vi "Read_SystemDevices_Values.vi"(8 "error in (no error)":errorcluster) -> (0 "error out":errorcluster)   [LabVIEW 2017]
doc: "reads all the values from the actual Instruments linked to the PrepLineObjects. It does not read the switches only the PGauges and TControllers etc etc.\n\nreads the current values of:\\\n- pressure\n- temp\n- temp set-point"
uses:
  Classes/PrepLineObject/PrepLineObject.lvclass
  Classes/Instrument/instrument.lvclass
  global variables.vi
  Classes/StatusLog/StatusLog.lvclass
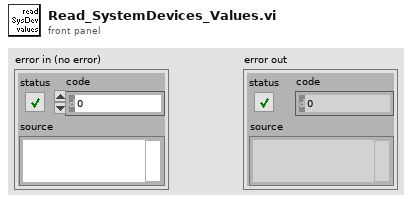
[diagram p1: front panel]
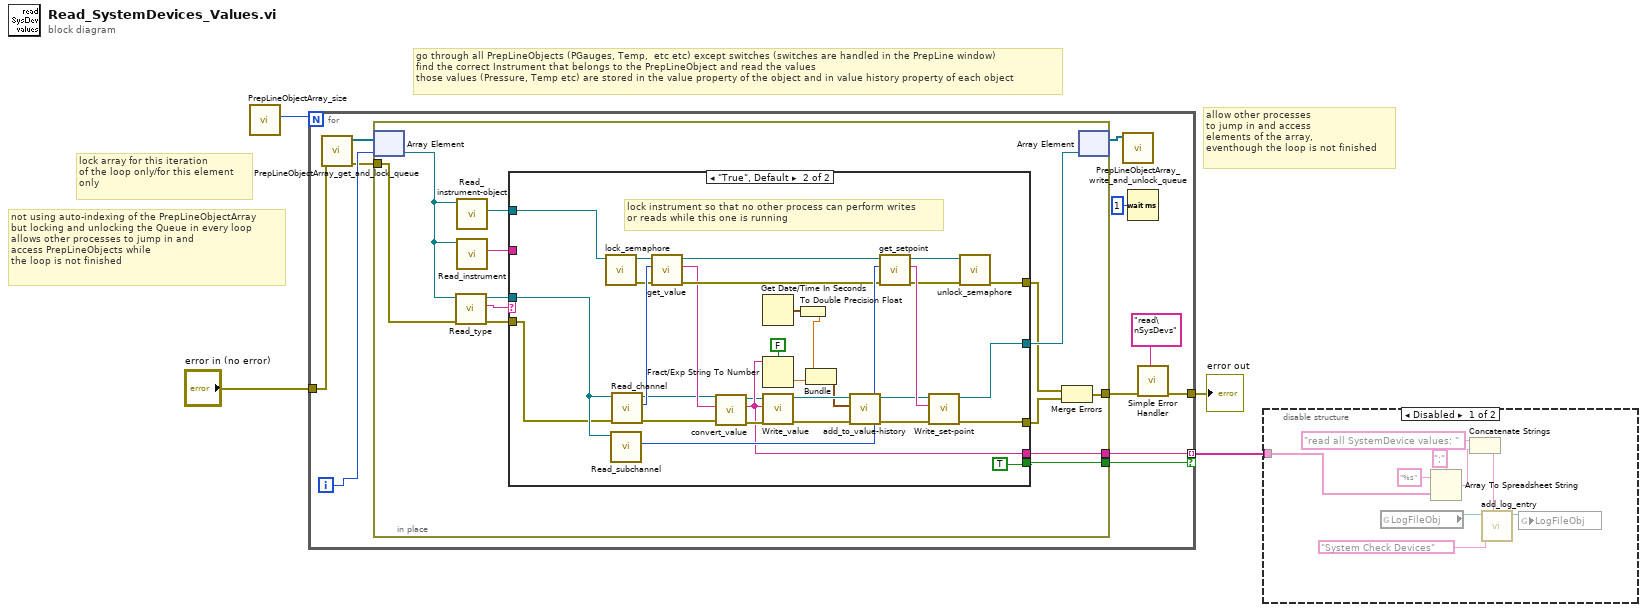
[diagram p0: block diagram]
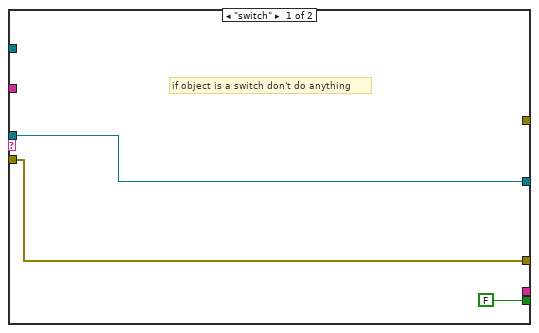
[diagram p3: hidden frame]
diagram:
  # "allow other processes\nto jump in and access\nelements of the array,\neventhough the loop is not finished"
  # "lock array for this iteration\nof the loop only/for this element\nonly"
  # "not using auto-indexing of the PrepLineObjectArray\nbut locking and unlocking the Queue in every loop\nallows other processes to jump in and\naccess PrepLineObjects while\nthe loop is not finished"
  # "go through all PrepLineObjects (PGauges, Temp,  etc etc) except switches (switches are handled in the PrepLine window)\nfind the correct Instrument that belongs to the PrepLineObject and read the values\nthose values (Pressure, Temp etc) are stored in the value property of the object and in value history property of each object"
  n1 = call "PrepLineObjectArray_size.vi"() -> ("size(s)"=w1:i32)  [unwired: 10 in, 1 out]
  n2 = for {
    N: w1 -> [_]
    tunnel: "error in (no error)" -> [w9]
    tunnel: [w15] -> w3 mode=indexing if=w14
    tunnel: [w6] -> w2
    i -> [w12]
    n3 = call "PrepLineObjectArray_get_and_lock_queue.vi"("error in (no error)"=w9) -> ("error out"=w8:errorcluster, "PrepLineObjects"=w13:refnum<class "PrepLineObject.lvclass">[])  [unwired: 9 in]
    n4 = in-place {
      in-place-border: [w25] -> w15
      in-place-border: [w24] -> w14
      in-place-border: [w16] -> w7
      in-place-border: w8 -> [w19]
      n5 = in-place-array #1(w13, w12) -> (w21:refnum<class "PrepLineObject.lvclass">)
      n6 = call-dynamic "Read_type.vi"("error in (no error)"=w19, "PrepLinePictureObjects in"=w21) -> ("error out"=w22:errorcluster, "type"=w27:string, "PrepLinePictureObjects out"=w26:refnum<class "PrepLineObject.lvclass">)  [unwired: 7 in]
      n7 = call-dynamic "Read_instrument-object.vi"("PrepLineObject in"=w21) -> ("instrument.lvclass"=w23:refnum<class "instrument.lvclass">)  [unwired: 8 in, 2 out]
      n8 = call-dynamic "Read_instrument.vi"("PrepLinePictureObjects in"=w21) -> ("instrument name"=w28:string)  [unwired: 7 in, 2 out]
      n9 = case shown="\"True\", Default" w27 {
        tunnel: [w31 w41] -> w20
        tunnel: w26 -> [w31 w50]
        tunnel: w28 -> [_ _]
        tunnel: [_ w34] -> w25
        tunnel: [FALSE TRUE] -> w24
        tunnel: w23 -> [_ w44]
        tunnel: w22 -> [w29 w43]
        tunnel: [w29 w40] -> w18
        tunnel: [_ w39] -> w17
        frame "switch" {
          # "if object is a switch don't do anything"
        }
        frame "True", Default {
          # "lock instrument so that no other process can perform writes\nor reads while this one is running"
          n10 = call-dynamic "lock_semaphore.vi"("instrument in"=w44) -> ("error out"=w53:errorcluster, "instrument out"=w54:refnum<class "instrument.lvclass">)  [unwired: 9 in]
          n11 = call-dynamic "Read_subchannel.vi"("PrepLineObject in"=w50) -> ("subchannel"=w48:u16)  [unwired: 8 in, 2 out]
          n12 = call-dynamic "Read_channel.vi"("error in (no error)"=w43, "PrepLineObject in"=w50) -> ("error out"=w36:errorcluster, "channel"=w56:u16, "PrepLineObject out"=w37:refnum<class "PrepLineObject.lvclass">)  [unwired: 7 in]
          n13 = call-dynamic "get_value.vi"("error in (no error)"=w53, "channel"=w56, "instrument in"=w54) -> ("error out"=w46:errorcluster, "value"=w38:string, "instrument out"=w52:refnum<class "instrument.lvclass">)  [unwired: 6 in]
          n14 = call-dynamic "convert_value.vi"("error in (no error)"=w36, "value in"=w38, "PrepLineObject in"=w37) -> ("error out"=w35:errorcluster, "converted value out"=w34:string, "PrepLineObject out"=w33:refnum<class "PrepLineObject.lvclass">)  [unwired: 6 in]
          n15 = Get Date/Time In Seconds() -> (seconds since 1Jan1904=w60:timestamp)
          n16 = Fract/Exp String To Number(use system decimal point (T)=FALSE, string=w34) -> (number=w57:dbl)  [unwired: 2 in, 1 out]
          n17 = call-dynamic "Write_value.vi"("error in (no error)"=w35, "value"=w34, "PrepLineObject in"=w33) -> ("error out"=w61:errorcluster, "PrepLineObject out"=w62:refnum<class "PrepLineObject.lvclass">)  [unwired: 7 in]
          n18 = To Double Precision Float(number=w60) -> (double precision float=w59:dbl)
          n19 = Bundle(w59, w57) -> (w58:cluster{dbl, dbl})  [unwired: 1 in]
          n20 = call-dynamic "add_to_value-history.vi"("error in (no error)"=w61, "Cluster"=w58, "PrepLineObject in"=w62) -> ("error out"=w42:errorcluster, "PrepLineObject out"=w49:refnum<class "PrepLineObject.lvclass">)  [unwired: 7 in]
          n21 = call-dynamic "get_setpoint.vi"("error in (no error)"=w46, "channel"=w48, "instrument in"=w52) -> ("error out"=w47:errorcluster, "setpoint"=w55:string, "instrument out"=w51:refnum<class "instrument.lvclass">)  [unwired: 6 in]
          n22 = call-dynamic "Write_set-point.vi"("error in (no error)"=w42, "set point"=w55, "PrepLineObject in"=w49) -> ("error out"=w40:errorcluster, "PrepLineObject out"=w41:refnum<class "PrepLineObject.lvclass">)  [unwired: 7 in]
          n23 = call-dynamic "unlock_semaphore.vi"("error in (no error)"=w47, "instrument in"=w51) -> ("error out"=w39:errorcluster)  [unwired: 8 in, 1 out]
        }
      }
      n24 = Merge Errors(w17, w18) -> (w16:errorcluster)
      n25 = in-place-array #1(w20) -> (w11:refnum<class "PrepLineObject.lvclass">[])  [unwired: 1 out]
    }
    n26 = call "PrepLineObjectArray_write_and_unlock_queue.vi"("PrepLineObjArray"=w11) -> ()  [unwired: 10 in, 1 out]
    n27 = Wait (ms)(milliseconds to wait=u32 1) -> ()  [unwired: 1 out]
    n28 = call <vilib>:"Simple Error Handler.vi"("error source (\" \")"="read\nSysDevs" ("error source (\" \")"), "error in (no error)"=w7) -> ("error out"=w6:errorcluster)  [unwired: 3 in, 4 out]
  }
  "error out" <- w2
  n29 = disable-structure shown="Disabled" {
    disable-tunnel: w3 -> [w68 _]
    frame Disabled {
      n30 = global read "global variables.vi" "LogFileObj"() -> (w70:refnum<class "StatusLog.lvclass">)
      n31 = Array To Spreadsheet String(delimiter (Tab)=";", array=w68, 3:"%s" ("format string")) -> (spreadsheet string=w66:string)
      n32 = Concatenate Strings("read all SystemDevice values: " ("format string"), w66) -> (w65:string)
      n33 = call-dynamic "add_log_entry.vi"("new entry"=w65, "log identifiers"="System Check Devices", "StatusLog in"=w70) -> ("StatusLog out"=w71:refnum<class "StatusLog.lvclass">)  [unwired: 5 in, 1 out]
      n34 = global write "global variables.vi" "LogFileObj"(w71) -> ()
    }
    frame Enabled {
    }
  }
